vi "pythonAllocateArrayUINT16.vi"(1 "size":i32) -> (0 "pointer":i64)   [LabVIEW 2017]
uses:
  dll/wormUtilities/x64/Release/wormUtilities.dll
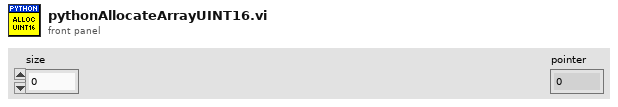
[diagram p1: front panel]
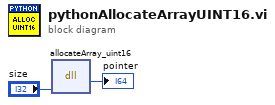
[diagram p0: block diagram]
diagram:
  n1 = dll-call lib="C:/Users/francesco/dev/pump-probe/dll/wormUtilities/x64/Release/wormUtilities.dll" fn="allocateArray_uint16"("size"="size") -> ("return type"=→"pointer":i64)  [unwired: 4 in, 2 out]
